vi "Set Parameters GUI.vi"(8 "error in (no error)":errorcluster, 11 "Lakeshore 218 in":refnum<class "Lakeshore 218.lvclass">) -> (0 "error out":errorcluster, 3 "Lakeshore 218 out":refnum<class "Lakeshore 218.lvclass">)   [LabVIEW 2022 SP3, in "Lakeshore 218.lvclass"]
uses:
  Lakeshore 218.lvclass
  Lakeshore 218.lvclass/Lakeshore 218.ctl
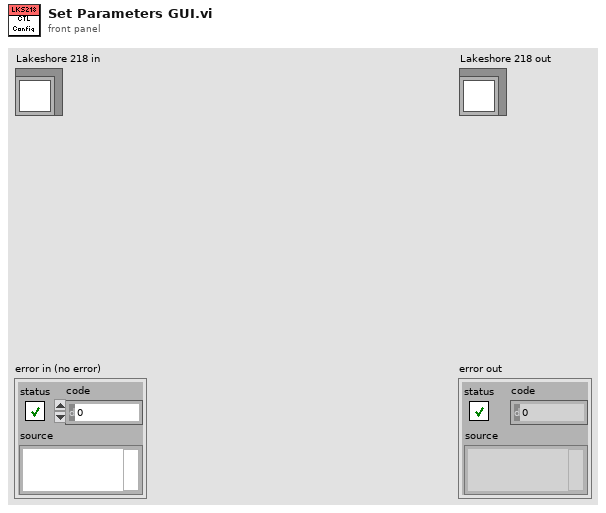
[diagram p1: front panel]
types:
  T1 = typedef "Lakeshore 218.lvclass/Lakeshore 218 cluster Settings.ctl" = cluster{"Port":refnum<visa-resource-name>, "Channel Names":string[], "Ch Enable":bool[]}
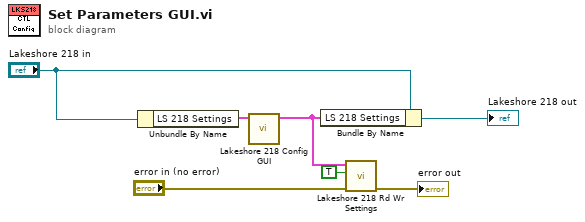
[diagram p0: block diagram]
diagram:
  n1 = Unbundle By Name("Lakeshore 218 in") -> ("LS 218 Settings"=w7:T1)
  n2 = call "Lakeshore 218 Config GUI.vi"("LS 218 Settings"=w7) -> ("Settings out"=w3:T1)  [unwired: 10 in]
  n3 = Bundle By Name(cluster="Lakeshore 218 in", "LS 218 Settings"=w3) -> (→"Lakeshore 218 out":refnum<class "Lakeshore 218.lvclass">)
  n4 = call "Lakeshore 218 Rd Wr Settings.vi"("error in (no error)"="error in (no error)", "Write? (F:Read)"=TRUE, "LS 218 Settings"=w3) -> ("error out"=→"error out":errorcluster)  [unwired: 7 in, 1 out]
